vi "Teleop.vi"(6 "Co_fifo":refnum<k33>, 7 "mechanism log":refnum<file>, 8 "drive log":refnum<file>, 9 "rt fifo":refnum<k33>, 10 "Match Info":T1={"Autonomous Elapsed Seconds"=0.0, "TeleOp Elapsed Seconds"=0.0, "Disabled Elapsed Seconds"=0.0, "Visited Autonomous"=FALSE, "Visited TeleOp"=FALSE, "Visited Disabled"=FALSE, "Autonomous Settings"={"Autonomous Style"=enum."Independent", "VI Refnum"=refnum}}, 11 "Call Context":T2) -> ()   [LabVIEW 2014]
doc: "This VI is called for each TeleOp packet received from the DS where the robot is not disabled. It is often used to read from the joysticks and update I/O or to update setpoints for timed control loops. It should complete and return within 20 milliseconds or it may miss DS packets."
uses:
  <vilib>/Rock Robotics/WPI/DriverStation/WPI_DriverStationDerivedRobotMode.ctl
  <vilib>/Rock Robotics/WPI/DriverStation/WPI_DriverStationMatch Info.ctl
  Lightning base/TeleopCmd.ctl
  Lightning base/CmdFlag.ctl
  Lightning base/Co-Pilot_game_control.ctl
  <vilib>/Rock Robotics/Network Tables/SD Read Boolean.vi
  <vilib>/Rock Robotics/Network Tables/SD Read Number.vi
panel:
  out "Sample Slider 0":dbl(slide) scale=0.0..5.0
  out "Sample Boolean 1":bool
  out "Sample Boolean 0":bool
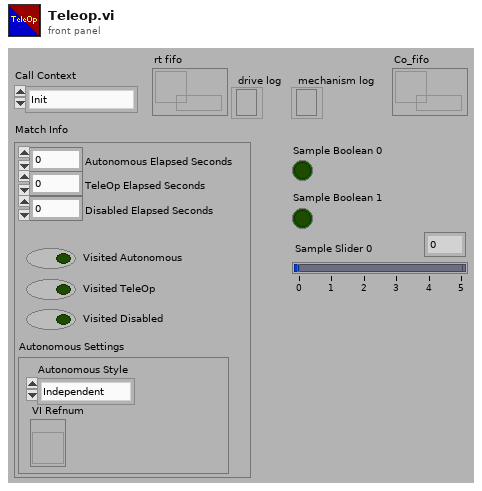
[diagram p1: front panel]
types:
  T1 = typedef "WPI_DriverStationMatch Info.ctl" = cluster{"Autonomous Elapsed Seconds":dbl, "TeleOp Elapsed Seconds":dbl, "Disabled Elapsed Seconds":dbl, "Visited Autonomous":bool, "Visited TeleOp":bool, "Visited Disabled":bool, "Autonomous Settings":cluster{"Autonomous Style":enum16{"Iterative", "Independent"}, "VI Refnum":refnum<vi>}}
  T2 = typedef "WPI_DriverStationDerivedRobotMode.ctl" = enum16{"Init", "Execute", "Stop"}
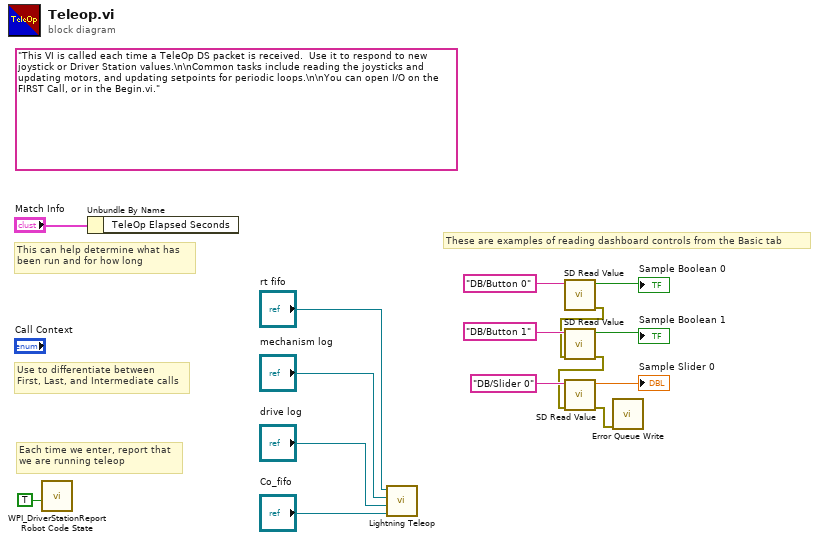
[diagram p0: block diagram]
diagram:
  (unwired) "This VI is called each time a TeleOp DS packet is received.  Use it to respond to new joystick or Driver Station values.\n\nCommon tasks include reading the joysticks and updating motors, and updating setpoints for periodic loops.\n\nYou can open I/O on the FIRST Call, or in the Begin.vi."
  # "These are examples of reading dashboard controls from the Basic tab"
  # "Each time we enter, report that\nwe are running teleop"
  # "Use to differentiate between\nFirst, Last, and Intermediate calls"
  # "This can help determine what has\nbeen run and for how long"
  n1 = call <vilib>:"WPI_DriverStationReport Robot Code State.vi"("TeleOp"=TRUE ("Autonomous")) -> ()  [unwired: 10 in, 1 out]
  n2 = Unbundle By Name("Match Info") -> ()  [unwired: 1 out]
  n3 = call "Lightning Teleop.vi"("Co_fifo"="Co_fifo", "drive log"="drive log", "mechanism log"="mechanism log", "rt fifo"="rt fifo") -> ()  [unwired: 8 in]
  n4 = call-poly <vilib>:"SD Read Value.vi"("Name"="DB/Button 0" ("refnum name")) -> ("error out"=w6:errorcluster, "Boolean"=→"Sample Boolean 0":bool)  [unwired: 8 in, 1 out]
  n5 = call-poly <vilib>:"SD Read Value.vi"("error in"=w6, "Name"="DB/Button 1" ("refnum name")) -> ("error out"=w5:errorcluster, "Boolean"=→"Sample Boolean 1":bool)  [unwired: 7 in, 1 out]
  n6 = call-poly <vilib>:"SD Read Value.vi"("error in"=w5, "Name"="DB/Slider 0" ("refnum name")) -> ("error out"=w4:errorcluster, "Numeric"=→"Sample Slider 0":dbl)  [unwired: 7 in, 1 out]
  n7 = call "Error Queue Write.vi"("error in (no error)"=w4) -> ()  [unwired: 11 in]
